vi "VariaveisGlobais.vi"() -> ()   [LabVIEW 2017]
panel:
  in  "IndicesDados":i32
  out "Velocimetro":dbl(knob) scale=0.06..60.0 scale format="%#_2g"
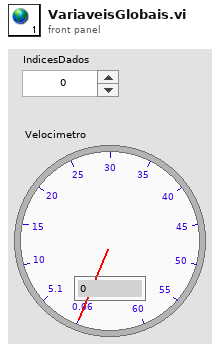
[diagram p1: front panel]
diagram:
